vi "Add Visible Tab.vi"(8 "error in (no error)":errorcluster, 10 "New Name":string, 11 "CIF_UI in":refnum<class "CIF_UI.lvclass">) -> (0 "error out":errorcluster)   [LabVIEW 2021, in "CIF_UI.lvclass"]
uses:
  CIF_UI.lvclass
  CIF_UI.lvclass/CIF_UI.ctl
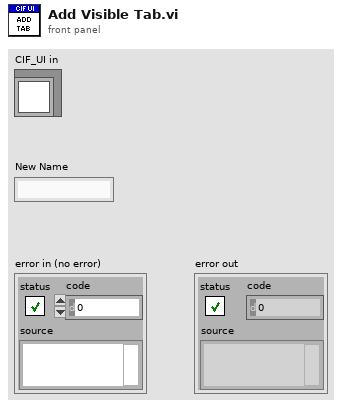
[diagram p1: front panel]
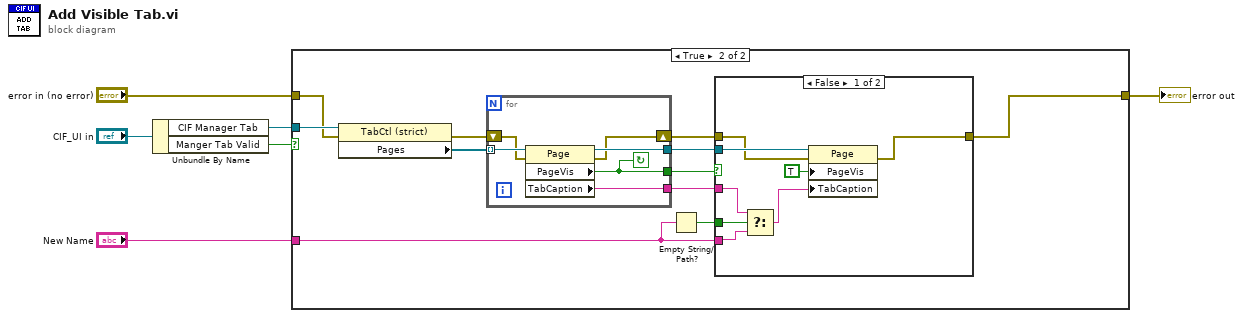
[diagram p0: block diagram]
diagram:
  n1 = Unbundle By Name("CIF_UI in") -> ("CIF Manager Tab"=w4:refnum<vi>, "Manger Tab Valid"=w5:bool)
  n2 = case shown="True" w5 {
    tunnel: w4 -> [_ w18]
    tunnel: "error in (no error)" -> [w7 w11]
    tunnel: [w7 w8] -> w2
    tunnel: "New Name" -> [_ w10]
    frame False {
    }
    frame True {
      n3 = property class="TabCtl (strict)"(reference=w18, error in=w11) -> (error out=w16:errorcluster, "Pages"=w17:refnum<vi>[])  [unwired: 1 out]
      n4 = for {
        tunnel: w17 -> [w33] mode=indexing
        tunnel: [w32] -> w14
        shift-right: [w30] -> w13
        shift-left: w16 -> [w31]
        tunnel: [w29] -> w15
        tunnel: [w28] -> w12
        stop <- w29 continue-if-true
        n5 = property class="Page"(reference=w33, error in=w31) -> (reference out=w32:refnum<vi>, error out=w30:errorcluster, "PageVis"=w29:bool, "TabCaption"=w28:string)
      }
      n6 = Empty String/Path?(string/path=w10) -> (empty?=w9:bool)
      n7 = case shown="False" w15 {
        tunnel: w14 -> [w26 _]
        tunnel: w13 -> [w25 w27]
        tunnel: w12 -> [w20 _]
        tunnel: [w23 w27] -> w8
        tunnel: w10 -> [w21 _]
        tunnel: w9 -> [w22 _]
        frame False {
          n8 = Select(t=w20, s=w22, f=w21) -> (s? t:f=w19:string)
          n9 = property class="Page"(reference=w26, error in=w25, "PageVis"=TRUE ("Page Visible"), "TabCaption"=w19) -> (error out=w23:errorcluster)  [unwired: 1 out]
        }
        frame True {
          # "No remaining tabs, could add warning"
        }
      }
    }
  }
  "error out" <- w2
